vi "ListIO.vi"(11 "Project":refnum<vi>) -> (0 "DI/O":string[](array[string]), 1 "AI":string[](array[string]), 2 "AO":string[](array[string]), 3 "DIOPORT":string[](array[string]), 4 "error out":errorcluster)   [LabVIEW 2024]
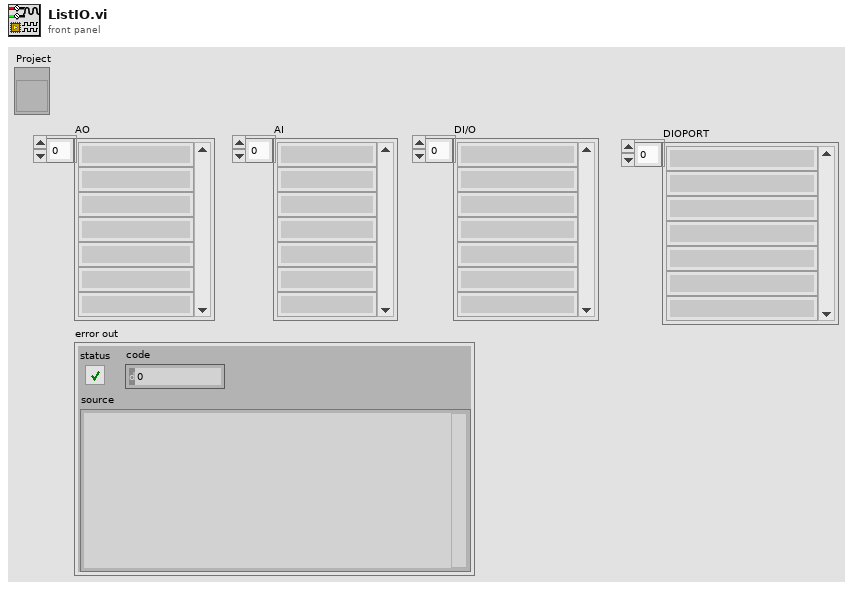
[diagram p1: front panel]
types:
  T1 = enum16{"open", "replace", "create", "open or create", "replace or create", "replace or create with confirmation"}
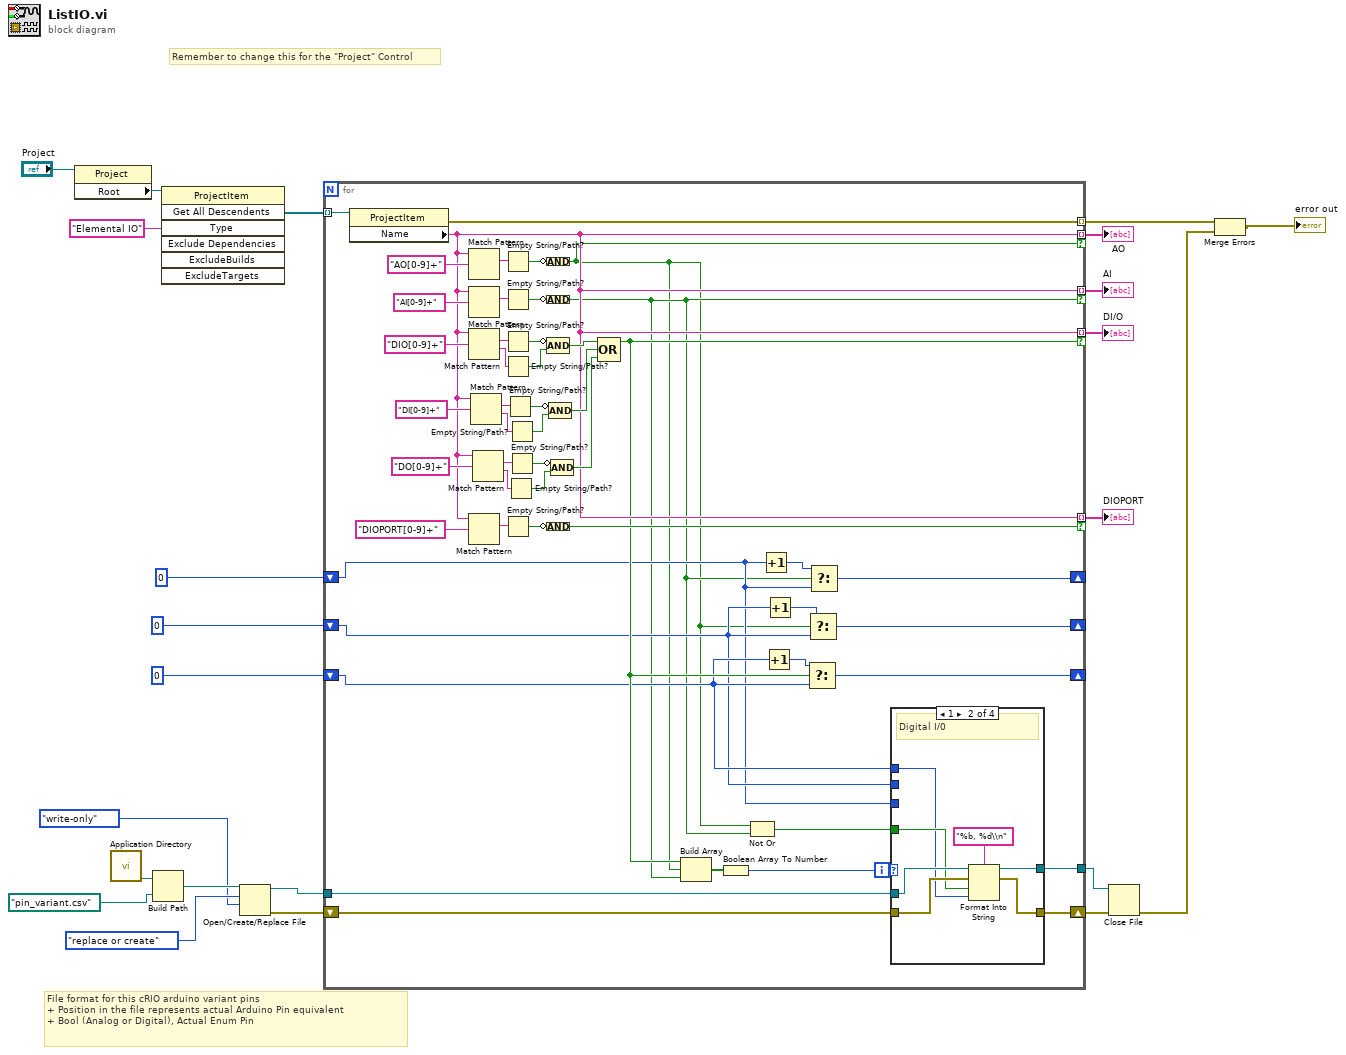
[diagram p0: block diagram]
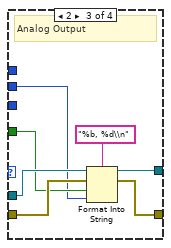
[diagram p3: hidden frame]
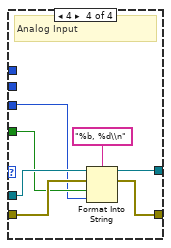
[diagram p4: hidden frame]
diagram:
  # "File format for this cRIO arduino variant pins\n+ Position in the file represents actual Arduino Pin equivalent\n+ Bool (Analog or Digital), Actual Enum Pin"
  # "Remember to change this for the \"Project\" Control"
  n1 = property class="Project"(reference="Project") -> ("Root"=w21:refnum<vi>)  [unwired: 1 in, 2 out]
  n2 = call <vilib>:"Application Directory.vi"() -> ("Application Directory"=w16:path)
  n3 = Build Path(base path=w16, name or relative path=path "pin_variant.csv") -> (appended path=w14:path)
  n4 = invoke class="ProjectItem" method="Get All Descendents"(reference=w21, "Type"="Elemental IO" ("Type String")) -> ("All Descendents"=w22:refnum<vi>[])  [unwired: 5 in, 6 out]
  n5 = Open/Create/Replace File(file path (use dialog)=w14, operation (0:open)=T1."replace or create", access (0:read/write)=enum16{"read/write", "read-only", "write-only"}."write-only") -> (refnum out=w8:refnum<file>, error out=w7:errorcluster)  [unwired: 3 in, 1 out]
  n6 = for {
    tunnel: w22 -> [w73] mode=indexing
    tunnel: [w49] -> w23 mode=indexing if=w29
    tunnel: [w72] -> w4 mode=indexing
    tunnel: [w49] -> w19 mode=indexing if=w30
    tunnel: [w49] -> w18 mode=indexing if=w36
    tunnel: [w49] -> w17 mode=indexing if=w58
    shift-right: [w42] -> _
    shift-left: 0 ("I/O element") -> [w31]
    shift-right: [w41] -> _
    shift-left: 0 ("I/O element") -> [w32]
    shift-right: [w40] -> _
    shift-left: 0 ("I/O element") -> [w33]
    tunnel: w8 -> [w28]
    tunnel: [w26] -> w1
    shift-right: [w25] -> w6
    shift-left: w7 -> [w27]
    n7 = property class="ProjectItem"(reference=w73) -> (error out=w72:errorcluster, "Name"=w49:string)  [unwired: 1 in, 1 out]
    n8 = Match Pattern(string=w49, regular expression="AO[0-9]+") -> (match substring=w70:string)  [unwired: 1 in, 3 out]
    n9 = Match Pattern(string=w49, regular expression="AI[0-9]+") -> (match substring=w67:string)  [unwired: 1 in, 3 out]
    n10 = Match Pattern(string=w49, regular expression="DIO[0-9]+") -> (match substring=w64:string, after substring=w44:string)  [unwired: 1 in, 2 out]
    n11 = Match Pattern(string=w49, regular expression="DIOPORT[0-9]+") -> (match substring=w60:string)  [unwired: 1 in, 3 out]
    n12 = Match Pattern(string=w49, regular expression="DI[0-9]+") -> (match substring=w56:string, after substring=w45:string)  [unwired: 1 in, 2 out]
    n13 = Match Pattern(string=w49, regular expression="DO[0-9]+") -> (match substring=w52:string, after substring=w48:string)  [unwired: 1 in, 2 out]
    n14 = Empty String/Path?(string/path=w70) -> (empty?=w69:bool)
    n15 = Empty String/Path?(string/path=w67) -> (empty?=w68:bool)
    n16 = Empty String/Path?(string/path=w64) -> (empty?=w63:bool)
    n17 = Empty String/Path?(string/path=w44) -> (empty?=w43:bool)
    n18 = Empty String/Path?(string/path=w60) -> (empty?=w61:bool)
    n19 = Empty String/Path?(string/path=w56) -> (empty?=w57:bool)
    n20 = Empty String/Path?(string/path=w48) -> (empty?=w47:bool)
    n21 = Empty String/Path?(string/path=w45) -> (empty?=w46:bool)
    n22 = Empty String/Path?(string/path=w52) -> (empty?=w51:bool)
    n23 = Compound Arithmetic op=AND(invert w69) -> (w29:bool)
    n24 = Compound Arithmetic op=AND(invert w68) -> (w30:bool)
    n25 = Compound Arithmetic op=AND(invert w63, w43) -> (w62:bool)
    n26 = Compound Arithmetic op=AND(invert w61) -> (w58:bool)
    n27 = Compound Arithmetic op=AND(invert w57, w46) -> (w54:bool)
    n28 = Compound Arithmetic op=AND(invert w51, w47) -> (w50:bool)
    n29 = Compound Arithmetic op=OR(w62, w54, w50) -> (w36:bool)
    n30 = Build Array(w36, w29, w30) -> (w35:bool[])
    n31 = Boolean Array To Number(Boolean array=w35) -> (number=w34:u32)
    n32 = Not Or(1:w30, 2:w29) -> (0:w24:bool)
    n33 = Increment(x=w31) -> (x+1=w39:i32)
    n34 = Increment(x=w33) -> (x+1=w37:i32)
    n35 = Increment(x=w32) -> (x+1=w38:i32)
    n36 = Select(t=w37, s=w36, f=w33) -> (s? t:f=w40:i32)
    n37 = Select(t=w38, s=w29, f=w32) -> (s? t:f=w41:i32)
    n38 = Select(t=w39, s=w30, f=w31) -> (s? t:f=w42:i32)
    n39 = case shown="1" w34 {
      tunnel: w33 -> [_ w76 _ _]
      tunnel: w32 -> [_ _ w83 _]
      tunnel: w31 -> [_ _ _ w90]
      tunnel: w28 -> [w75 w82 w89 w96]
      tunnel: w27 -> [w74 w81 w88 w95]
      tunnel: [w75 w80 w87 w94] -> w26
      tunnel: [w74 w79 w86 w93] -> w25
      tunnel: w24 -> [_ w78 w85 w92]
      frame 0, Default {
        # "Do not record (Invalid Element I/O for Arduino)"
      }
      frame 1 {
        # "Digital I/0"
        n40 = Format Into String(format string="%b, %d\\n", initial string=w82, error in=w81, w78, w76) -> (resulting string=w80:refnum<file>, error out=w79:errorcluster)
      }
      frame 2 {
        # "Analog Output"
        n41 = Format Into String(format string="%b, %d\\n", initial string=w89, error in=w88, w85, w83) -> (resulting string=w87:refnum<file>, error out=w86:errorcluster)
      }
      frame 4 {
        # "Analog Input"
        n42 = Format Into String(format string="%b, %d\\n", initial string=w96, error in=w95, w92, w90) -> (resulting string=w94:refnum<file>, error out=w93:errorcluster)
      }
    }
  }
  "AO" <- w23
  "AI" <- w19
  "DI/O" <- w18
  "DIOPORT" <- w17
  n43 = Close File(refnum=w1, error in=w6) -> (error out=w3:errorcluster)  [unwired: 1 out]
  n44 = Merge Errors(w4, w3) -> (→"error out":errorcluster)
